vi "Subvi counter U32.vi"(8 "Reset":bool, 9 "+1":bool) -> (1 "Count":u32)   [LabVIEW 2017]
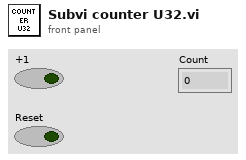
[diagram p1: front panel]
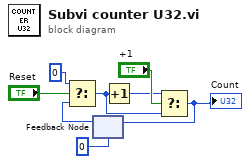
[diagram p0: block diagram]
diagram:
  n1 = feedback #1(u32 0) -> (w5:u32)
  n2 = Select(t=u32 0, s="Reset", f=w5) -> (s? t:f=w1:u32)
  n3 = Increment(x=w1) -> (x+1=w3:u32)
  n4 = Select(t=w3, s="+1", f=w1) -> (s? t:f=w7:u32)
  "Count" <- w7
  n5 = feedback-in #1(w7) -> ()
